vi "XNET Bus Monitor Example.vi"() -> ()   [LabVIEW 2025, in "XNET Bus Monitor Client.lvlib"]
uses:
  XNET Bus Monitor Client.lvlib
  Types/GUI.StateVariables.ctl
  Types/StreamEngine.CmdQueueData.ctl
  Types/StreamEngine.Parameters.ctl
  <vilib>/Utility/miscctls.llb/LVRowAndColumnUnsignedTypeDef.ctl
  Types/StreamEngine.CmdQueueData.Cmd.ctl
  Types/StreamEngine.QueueRefs.ctl
  Types/GUI.Controls.Refs.ctl
  bus_monitor_client/RPC Messages/ni_bus_monitor_api_Frame.ctl
  bus_monitor_client/bus_monitor_client.lvlib
  <vilib>/gRPC/LabVIEW gRPC Library/Shared/grpcId.ctl
  <vilib>/gRPC/LabVIEW gRPC Library/grpc-lvsupport-release.lvlib
  bus_monitor_client/RPC Messages/ni_bus_monitor_api_FrameFilter.ctl
  bus_monitor_client/RPC Messages/ni_bus_monitor_api_DirectionFilter.ctl
  bus_monitor_client/RPC Messages/ni_bus_monitor_api_FilterInfo.ctl
  bus_monitor_client/RPC Messages/ni_bus_monitor_api_SetStreamingFilterRequest.ctl
  bus_monitor_client/RPC Messages/ni_bus_monitor_api_PassThruRequest.ctl
  Types/gRPC.ConnectionInfo.ctl
  Types/StreamEngine.State.ctl
  Types/SubProcessEngine.CmdQueueData.ctl
  Types/SubProcessEngine.CmdQueueData.Cmd.ctl
  Types/SubProcessEngine.State.ctl
  bus_monitor_client/RPC Messages/ni_bus_monitor_api_ErrorInfo.ctl
  bus_monitor_client/RPC Messages/ni_bus_monitor_api_StreamBusReply.ctl
  Types/StreamEngine.CmdQueueData.InitialSettings.ctl
  Types/SubProcessEngine.CmdQueueData.Publish.ctl
  Types/SubProcessEngine.QueueRefs.ctl
  bus_monitor_client/RPC Messages/ni_bus_monitor_api_Session.ctl
  bus_monitor_client/RPC Messages/ni_bus_monitor_api_ResetStreamingFilterRequest.ctl
  bus_monitor_client/RPC Messages/ni_bus_monitor_api_GetStreamingFilterRequest.ctl
  bus_monitor_client/RPC Messages/ni_bus_monitor_api_StopProcessRequest.ctl
  bus_monitor_client/RPC Messages/ni_bus_monitor_api_LastCommError.ctl
  bus_monitor_client/RPC Messages/ni_bus_monitor_api_CommState.ctl
  bus_monitor_client/RPC Messages/ni_bus_monitor_api_CanCommState.ctl
panel:
  out "error out":errorcluster
  out "Device":string
  in  "Tab Control":enum32{"Bus Stream", "RAW"}(tab)
  out "Log Status":string
  in  "Direction Filter":T1
  in  "Type Filter":T2
  in  "Reset Filter":bool
  in  "Host Filter":bool
  in  "Filter IDs":string caption="Filter IDs (format = x<ID>, comma separated, ID x0 = Bus Error)"
  in  "Clear History":bool
  out "Table Control":string[][](table)
  in  "Sort By ID":bool
  out "Stream Connected":bool
  out "Bus Status":string
  in  "Log":bool
  in  "Pause":bool
  in  "Extended?":bool
  in  "Identifier":u32 format="%x"
  in  "Raw Bytes":u8[](array[numeric])
  in  "Type":T3(ring)
  out "Error":errorcluster
  in  "Clear Raw":bool
  in  "Send Raw":bool
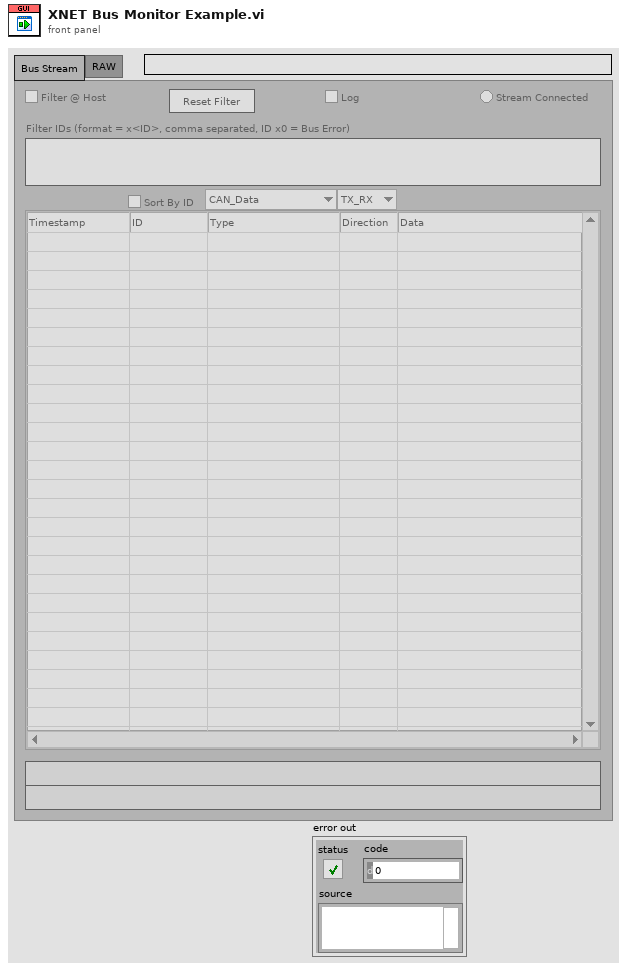
[diagram p1: front panel]
types:
  T1 = typedef "bus_monitor_client.lvlib/ni_bus_monitor_api_DirectionFilter.ctl" = enum32{"TX_RX", "RX", "TX"}
  T2 = typedef "bus_monitor_client.lvlib/ni_bus_monitor_api_FrameFilter.ctl" = enum32{"CAN_Data", "CAN_Remote", "CAN_Bus_Error", "CAN_2_Data", "CAN_FD_Data", "CAN_FD_BRS_Data", "J1939_Data", "Delay", "Log_Trigger", "Start_Trigger", "All"}
  T3 = enum16{"CAN Data", "CAN Remote", "CAN Bus Error", "CAN 2.0 Data", "CAN FD Data", "CAN FD+BRS Data", "J1939 Data", "Delay", "Log Trigger", "Start Trigger"}
  T4 = typedef "XNET Bus Monitor Client.lvlib/StreamEngine.CmdQueueData.InitialSettings.ctl" = cluster{"gRPC ID":T5, "Session":T6, "Project Folder":path}
  T5 = typedef "grpc-lvsupport-release.lvlib/grpcId.ctl" = u64
  T6 = typedef "bus_monitor_client.lvlib/ni_bus_monitor_api_Session.ctl" = cluster{"name":string, "session_uid":string}
  T7 = typedef "XNET Bus Monitor Client.lvlib/SubProcessEngine.State.ctl" = enum8{"Idle", "Arm", "Process", "Stop", "Exit"}
  T8 = typedef "XNET Bus Monitor Client.lvlib/StreamEngine.State.ctl" = enum8{"Wait", "Start Stream", "Read Stream", "Stop Stream", "Exit"}
  T9 = typedef "XNET Bus Monitor Client.lvlib/GUI.StateVariables.ctl" = cluster{"UI.Refs":T10, "Connected?":bool, "Stream.Qs":T11, "Log Path":path, "gRPC Info":T13}
  T10 = typedef "XNET Bus Monitor Client.lvlib/GUI.Controls.Refs.ctl" = cluster{"Device":refnum<vi>, "Pause":refnum<vi>, "Table Control":refnum<vi>, "Sort By ID":refnum<vi>, "Streaming Connected":refnum<vi>, "Bus Status":refnum<vi>, "Direction Filter":refnum<vi>, "Type Filter":refnum<vi>, "Clear History":refnum<vi>, "Filter IDs":refnum<vi>, "Filter Location":refnum<vi>, "Reset Filter":refnum<vi>, "Log":refnum<vi>, "Type":refnum<vi>, "Extended?":refnum<vi>, "Identifier":refnum<vi>, "Raw Bytes":refnum<vi>, "Send Raw":refnum<vi>, "Clear Raw":refnum<vi>, "Raw Error":refnum<vi>, "Log Status":refnum<vi>}
  T11 = typedef "XNET Bus Monitor Client.lvlib/StreamEngine.QueueRefs.ctl" = cluster{"Cmd":refnum<queue>, "SubProcesses":T12}
  T12 = typedef "XNET Bus Monitor Client.lvlib/SubProcessEngine.QueueRefs.ctl" = cluster{"Process":refnum<queue>, "Log":refnum<queue>}
  T13 = typedef "XNET Bus Monitor Client.lvlib/gRPC.ConnectionInfo.ctl" = cluster{"IP Address":string, "Service Name":string, "Found Port":u64, "ID":T5, "Session":T6}
  T14 = typedef "bus_monitor_client.lvlib/ni_bus_monitor_api_StopProcessRequest.ctl" = cluster{"session":T6}
  T15 = typedef "bus_monitor_client.lvlib/ni_bus_monitor_api_PassThruRequest.ctl" = cluster{"session":T6, "frame":T16}
  T16 = typedef "bus_monitor_client.lvlib/ni_bus_monitor_api_Frame.ctl" = cluster{"timestamp":dbl, "payload":u8[], "identifier":u32, "frame_type":u32, "extended":bool, "echo":bool}
  T17 = typedef "bus_monitor_client.lvlib/ni_bus_monitor_api_SetStreamingFilterRequest.ctl" = cluster{"session":T6, "filter_info":T18}
  T18 = typedef "bus_monitor_client.lvlib/ni_bus_monitor_api_FilterInfo.ctl" = cluster{"filter_ids":u32[], "direction_filter":T1, "frame_filter":T2}
  T19 = typedef "bus_monitor_client.lvlib/ni_bus_monitor_api_ResetStreamingFilterRequest.ctl" = cluster{"session":T6}
  T20 = typedef "bus_monitor_client.lvlib/ni_bus_monitor_api_GetStreamingFilterRequest.ctl" = cluster{"session":T6}
  T21 = typedef "LVRowAndColumnUnsignedTypeDef.ctl" = cluster{"Row":u32, "Column":u32}
  T22 = typedef "bus_monitor_client.lvlib/ni_bus_monitor_api_StopProcessReply.ctl" = cluster{"stopped":bool, "error":T23}
  T23 = typedef "bus_monitor_client.lvlib/ni_bus_monitor_api_ErrorInfo.ctl" = errorcluster
  T24 = enum8{"Enabled", "Disabled", "Disabled and Grayed Out"}
  T25 = typedef "bus_monitor_client.lvlib/ni_bus_monitor_api_PassThruReply.ctl" = cluster{"error":T23}
  T26 = typedef "bus_monitor_client.lvlib/ni_bus_monitor_api_SetStreamingFilterReply.ctl" = cluster{"error":T23}
  T27 = typedef "bus_monitor_client.lvlib/ni_bus_monitor_api_ResetStreamingFilterReply.ctl" = cluster{"filter_info":T18, "error":T23}
  T28 = typedef "bus_monitor_client.lvlib/ni_bus_monitor_api_GetStreamingFilterReply.ctl" = cluster{"filter_info":T18, "error":T23}
  T29 = typedef "XNET Bus Monitor Client.lvlib/SubProcessEngine.CmdQueueData.Publish.ctl" = cluster{"Response Data":T30, "Success":bool}
  T30 = typedef "bus_monitor_client.lvlib/ni_bus_monitor_api_StreamBusReply.ctl" = cluster{"can_comm_state":T31, "frame":T16[], "error":T23}
  T31 = typedef "bus_monitor_client.lvlib/ni_bus_monitor_api_CanCommState.ctl" = cluster{"fault_code":i32, "fault":bool, "comm_state":T32, "last_comm_error":T33, "receive_error_counter":u32, "transmit_error_counter":u32, "transceiver_error":bool, "sleep":bool}
  T32 = typedef "bus_monitor_client.lvlib/ni_bus_monitor_api_CommState.ctl" = enum32{"Error_Active", "Error_Passive", "Bus_Off", "Init"}
  T33 = typedef "bus_monitor_client.lvlib/ni_bus_monitor_api_LastCommError.ctl" = enum32{"None", "Stuff", "Form", "ACK", "Bit1", "Bit0", "CRC"}
  T34 = typedef "XNET Bus Monitor Client.lvlib/SubProcessEngine.CmdQueueData.ctl" = cluster{"Cmd":T35, "Parameters":variant}
  T35 = typedef "XNET Bus Monitor Client.lvlib/SubProcessEngine.CmdQueueData.Cmd.ctl" = enum16{"Arm", "Publish", "Stop", "Exit"}
  T36 = typedef "XNET Bus Monitor Client.lvlib/StreamEngine.Parameters.ctl" = cluster{"Host Filter":bool, "Filter Parameters":T18, "Sort By ID":bool, "Pause":bool, "Clear History":bool}
  T37 = typedef "XNET Bus Monitor Client.lvlib/StreamEngine.CmdQueueData.ctl" = cluster{"Cmd":T38, "Parameters":variant}
  T38 = typedef "XNET Bus Monitor Client.lvlib/StreamEngine.CmdQueueData.Cmd.ctl" = enum8{"Start Stream", "Stop Stream", "Exit"}
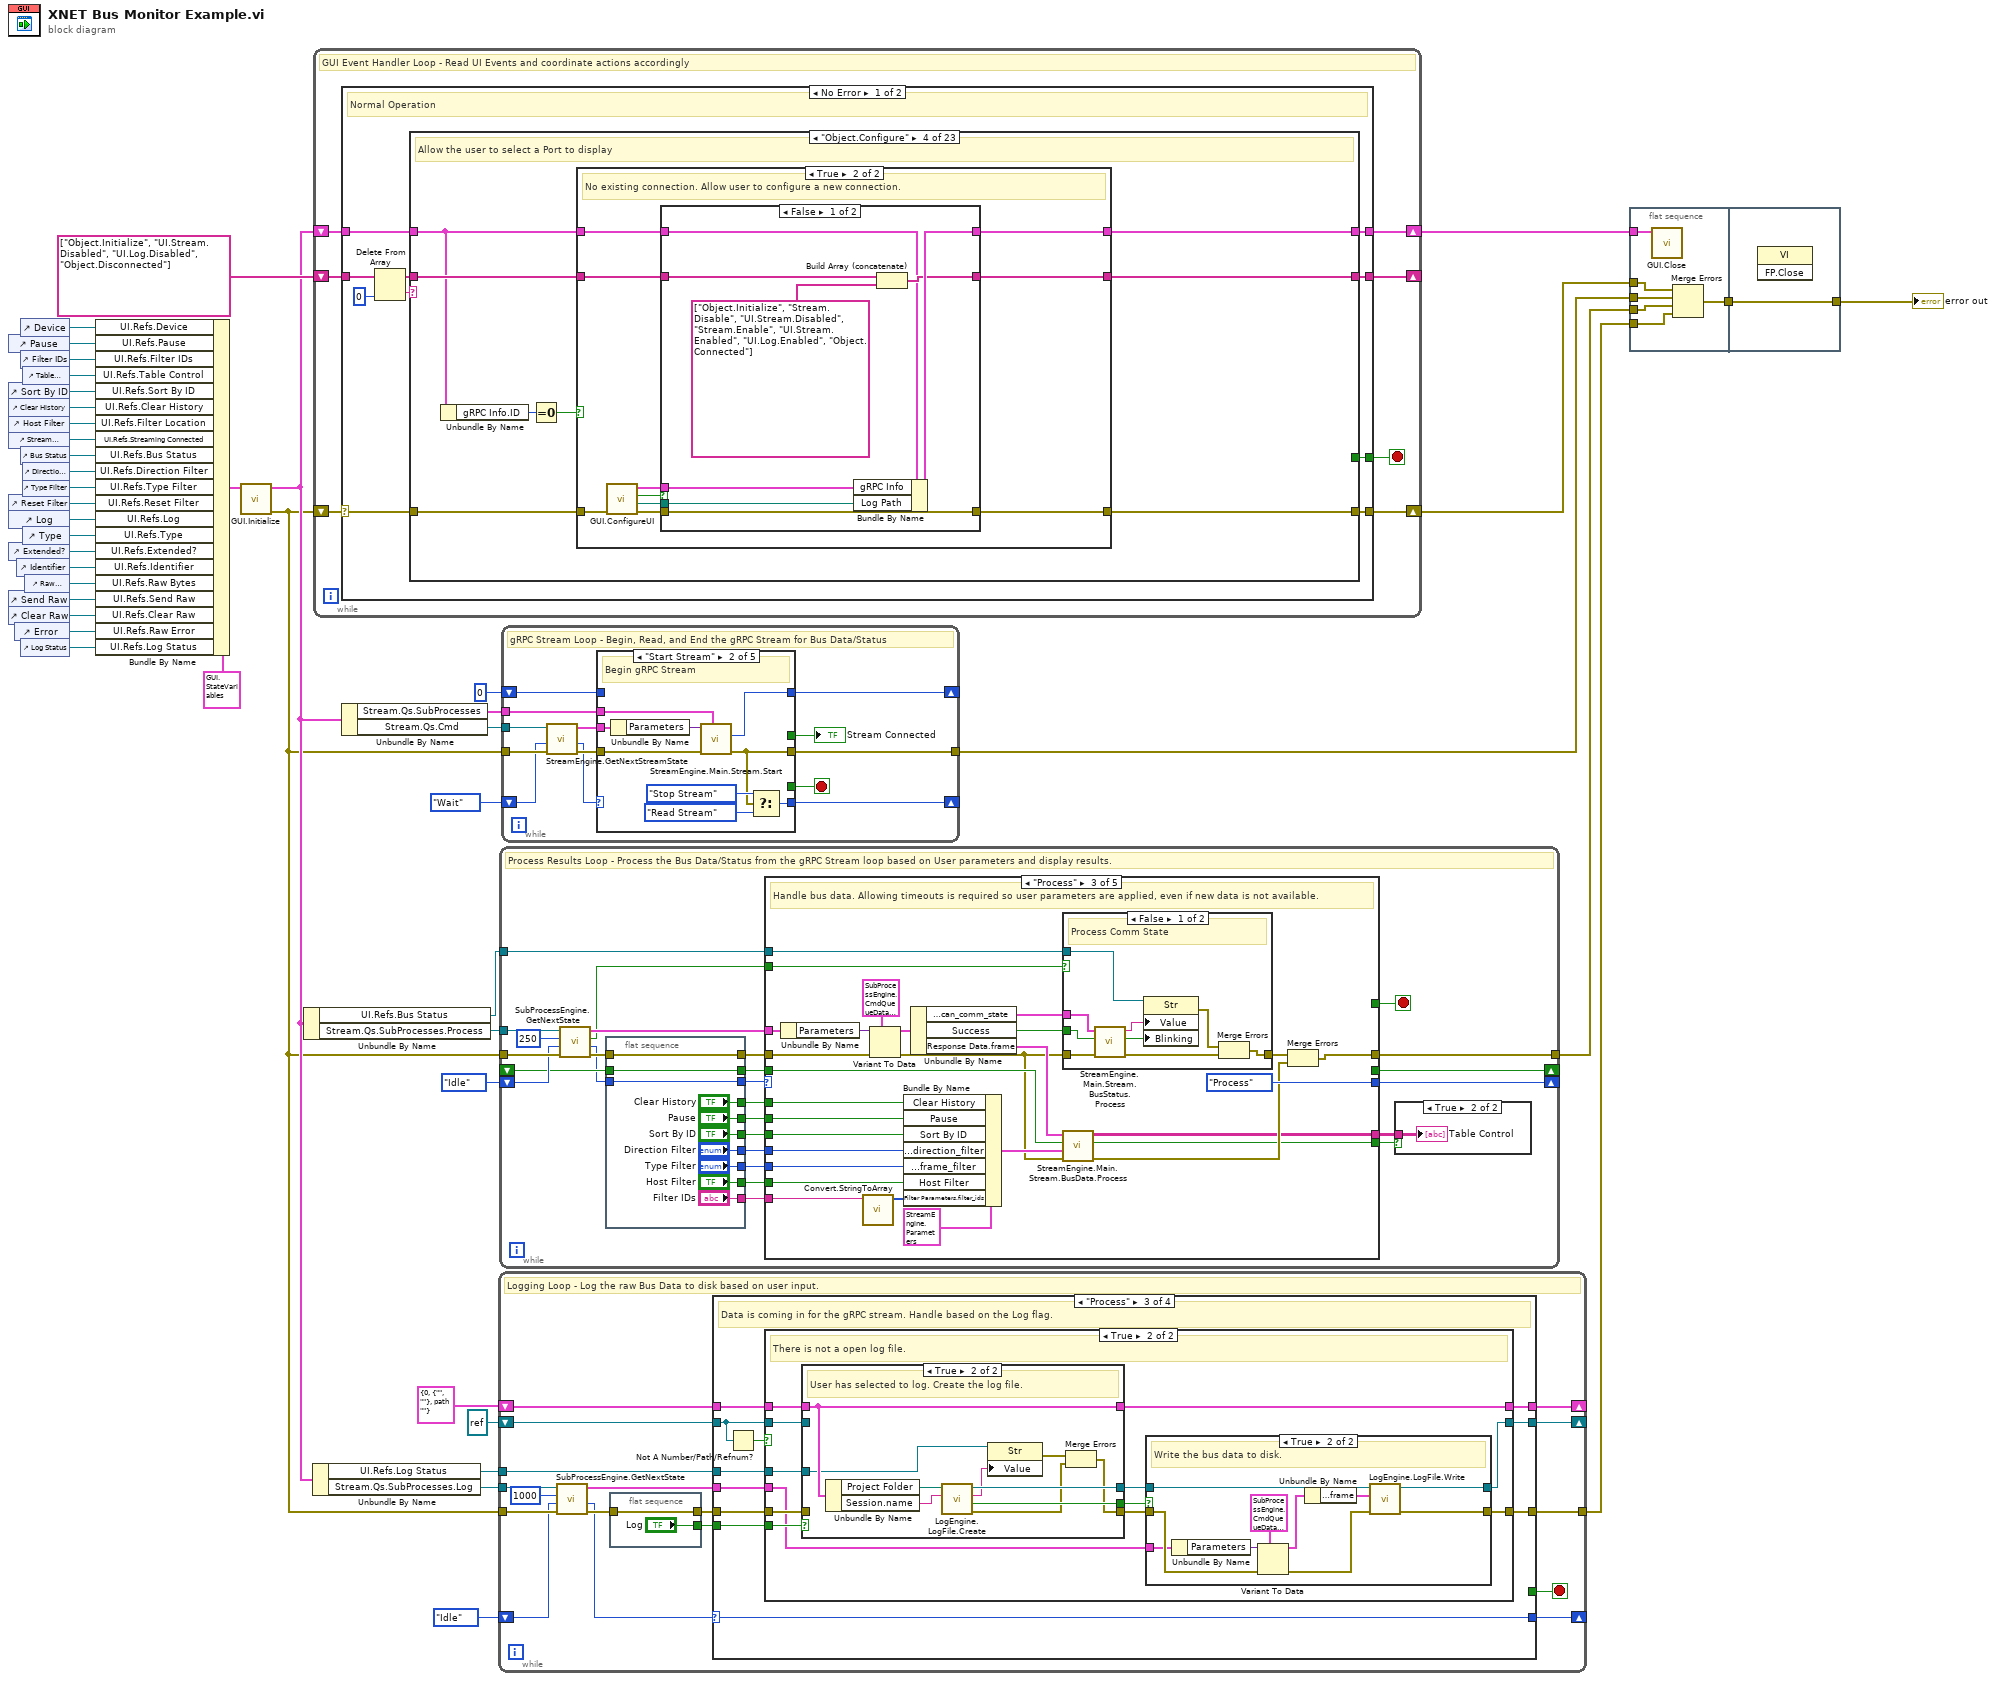
[diagram p0: block diagram]
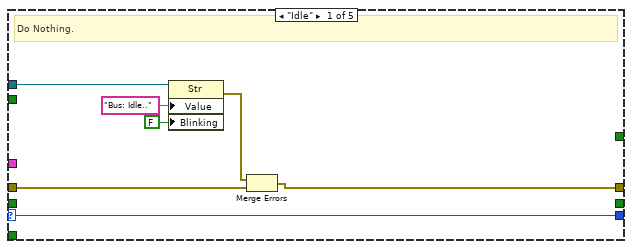
[diagram p3: hidden frame]
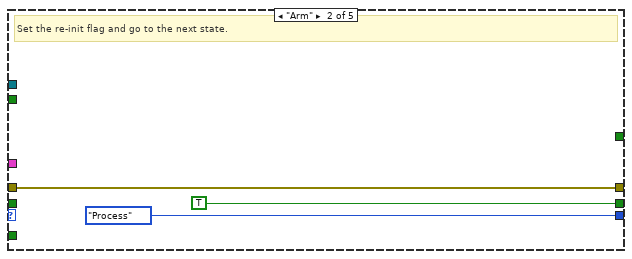
[diagram p4: hidden frame]
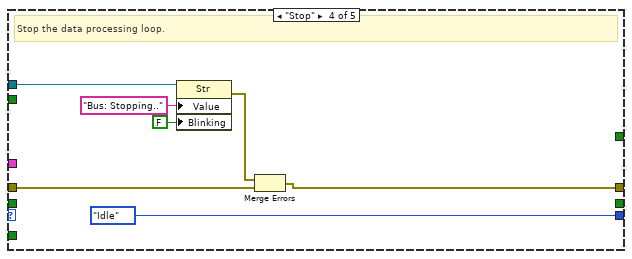
[diagram p6: hidden frame]
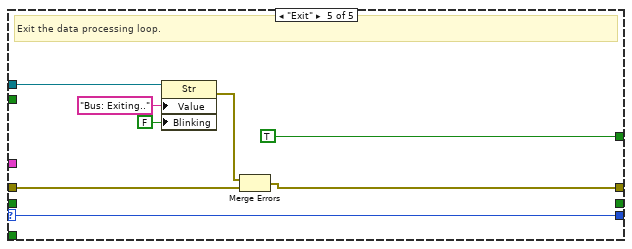
[diagram p7: hidden frame]
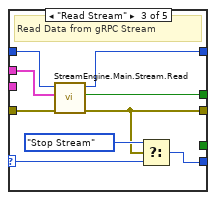
[diagram p9: hidden frame]
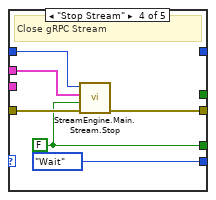
[diagram p10: hidden frame]
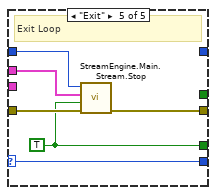
[diagram p11: hidden frame]
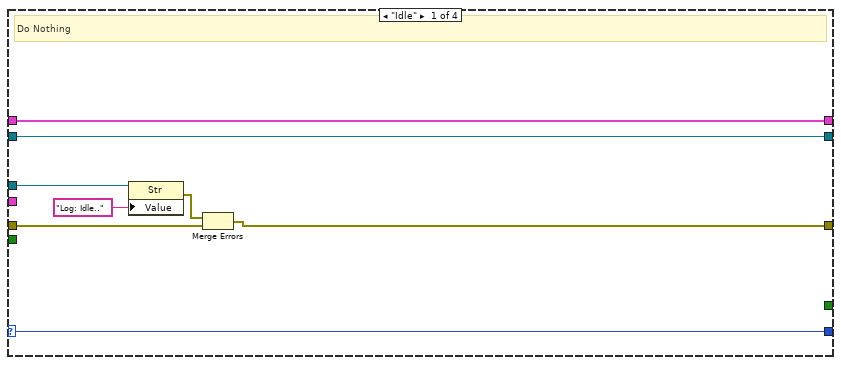
[diagram p12: hidden frame]
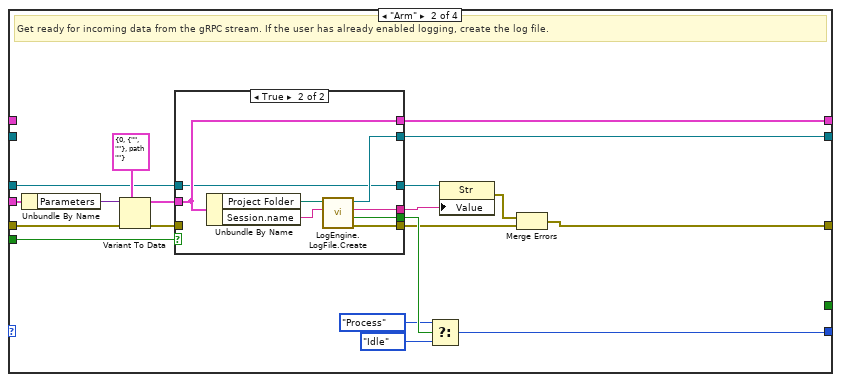
[diagram p13: hidden frame]
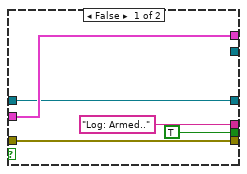
[diagram p14: hidden frame]
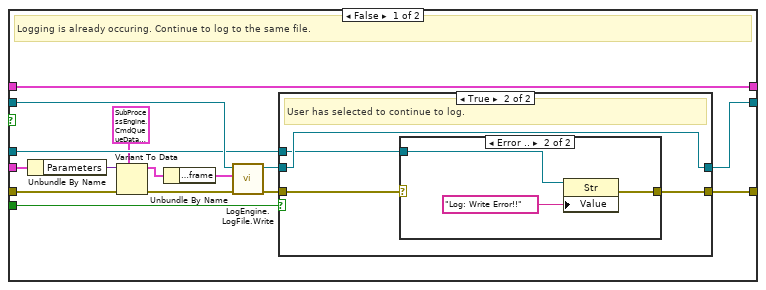
[diagram p15: hidden frame]
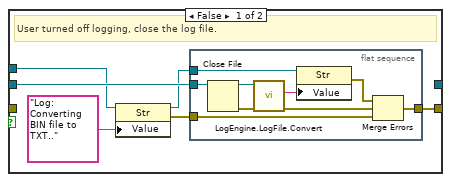
[diagram p16: hidden frame]
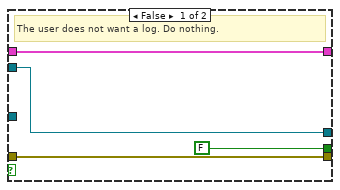
[diagram p19: hidden frame]
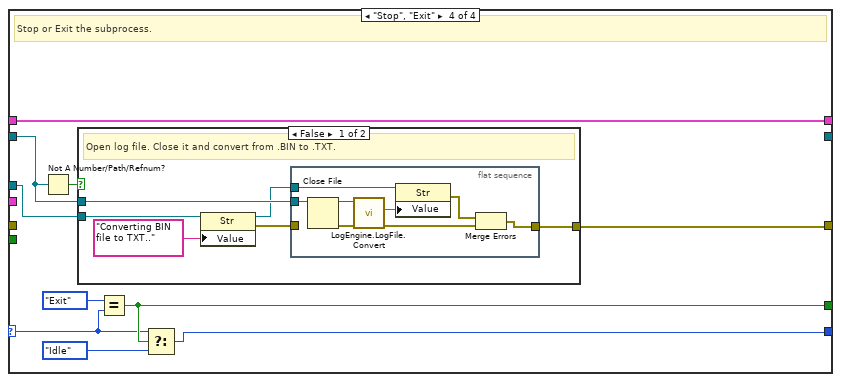
[diagram p20: hidden frame]
diagram:
  n1 = control-ref of="Pause"() -> (w22:refnum<vi>)
  n2 = control-ref of="Sort By ID"() -> (w41:refnum<vi>)
  n3 = control-ref of="Clear History"() -> (w37:refnum<vi>)
  n4 = control-ref of="Host Filter"() -> (w36:refnum<vi>)
  n5 = control-ref of="Stream Connected"() -> (w40:refnum<vi>)
  n6 = control-ref of="Reset Filter"() -> (w35:refnum<vi>)
  n7 = control-ref of="Log"() -> (w34:refnum<vi>)
  n8 = control-ref of="Extended?"() -> (w30:refnum<vi>)
  n9 = control-ref of="Send Raw"() -> (w27:refnum<vi>)
  n10 = control-ref of="Clear Raw"() -> (w28:refnum<vi>)
  n11 = control-ref of="Error"() -> (w29:refnum<vi>)
  n12 = control-ref of="Identifier"() -> (w31:refnum<vi>)
  n13 = control-ref of="Device"() -> (w24:refnum<vi>)
  n14 = control-ref of="Filter IDs"() -> (w38:refnum<vi>)
  n15 = control-ref of="Bus Status"() -> (w39:refnum<vi>)
  n16 = control-ref of="Log Status"() -> (w6:refnum<vi>)
  n17 = control-ref of="Table Control"() -> (w42:refnum<vi>)
  n18 = control-ref of="Direction Filter"() -> (w25:refnum<vi>)
  n19 = control-ref of="Type Filter"() -> (w26:refnum<vi>)
  n20 = control-ref of="Type"() -> (w33:refnum<vi>)
  n21 = control-ref of="Raw Bytes"() -> (w32:refnum<vi>)
  n22 = Bundle By Name(cluster=T9 {"UI.Refs"={"Device"=refnum, "Pause"=refnum, "Table Control"=refnum, "Sort By ID"=refnum, "Streaming Connected"=refnum, "Bus Status"=refnum, "Direction Filter"=refnum, "Type Filter"=refnum, "Clear History"=refnum, "Filter IDs"=refnum, "Filter Location"=refnum, "Reset Filter"=refnum, "Log"=refnum, "Type"=refnum, "Extended?"=refnum, "Identifier"=refnum, "Raw Bytes"=refnum, "Send Raw"=refnum, "Clear Raw"=refnum, "Raw Error"=refnum, "Log Status"=refnum}, "Connected?"=FALSE, "Stream.Qs"={"Cmd"=refnum, "SubProcesses"={"Process"=refnum, "Log"=refnum}}, "Log Path"=path "", "gRPC Info"={"IP Address"="", "Service Name"="", "Found Port"=0, "ID"=0, "Session"={"name"="", "session_uid"=""}}}, "UI.Refs.Device"=w24, "UI.Refs.Pause"=w22, "UI.Refs.Filter IDs"=w38, "UI.Refs.Table Control"=w42, "UI.Refs.Sort By ID"=w41, "UI.Refs.Clear History"=w37, "UI.Refs.Filter Location"=w36, "UI.Refs.Streaming Connected"=w40, "UI.Refs.Bus Status"=w39, "UI.Refs.Direction Filter"=w25, "UI.Refs.Type Filter"=w26, "UI.Refs.Reset Filter"=w35, "UI.Refs.Log"=w34, "UI.Refs.Type"=w33, "UI.Refs.Extended?"=w30, "UI.Refs.Identifier"=w31, "UI.Refs.Raw Bytes"=w32, "UI.Refs.Send Raw"=w27, "UI.Refs.Clear Raw"=w28, "UI.Refs.Raw Error"=w29, "UI.Refs.Log Status"=w6) -> (w23:T9)
  n23 = call "GUI.Initialize.vi"("State Variables in"=w23) -> ("error out"=w10:errorcluster, "State Variables out"=w13:T9)  [unwired: 9 in]
  n24 = Unbundle By Name(w13) -> ("UI.Refs.Bus Status"=w17:refnum<vi>, "Stream.Qs.SubProcesses.Process"=w18:refnum<queue>)
  n25 = Unbundle By Name(w13) -> ("UI.Refs.Log Status"=w5:refnum<vi>, "Stream.Qs.SubProcesses.Log"=w12:refnum<queue>)
  n26 = while {
    shift-right: [w50] -> _
    shift-left: string[] ["Object.Initialize", "UI.Stream.Disabled", "UI.Log.Disabled", "Object.Disconnected"] -> [w51]
    shift-right: [w48] -> w43
    shift-left: w13 -> [w47]
    shift-right: [w49] -> w8
    shift-left: w10 -> [w46]
    stop <- w52 stop-if-true
    # "GUI Event Handler Loop - Read UI Events and coordinate actions accordingly"
    n27 = case shown="No Error" w46 {
      selector: w46 -> [w53 w415]
      tunnel: [w62 _] -> w52
      tunnel: w51 -> [w60 w419]
      tunnel: [w57 w419] -> w50
      tunnel: [w56 w416] -> w49
      tunnel: [w55 w418] -> w48
      tunnel: w47 -> [w54 w418]
      frame No Error {
        # "Normal Operation"
        n28 = Delete From Array(array=w60, index=0) -> (deleted portion=w59:string, array with subset deleted=w58:string[])  [unwired: 1 in]
        n29 = case shown="\"Object.Configure\"" w59 {
          tunnel: [_ _ _ _ _ _ _ _ _ _ _ _ _ _ _ _ _ _ _ _ _ FALSE TRUE] -> w62
          tunnel: [w65 w71 w170 w178 w227 w236 w262 w264 w271 w285 w298 w311 w329 w333 w340 w354 w364 w379 w393 w399 w404 w410 w414] -> w57
          tunnel: w53 -> [w64 w69 w166 w176 w224 w233 w260 w266 w269 w282 w296 w308 w328 w332 w339 w352 w362 w377 w391 w394 w400 w407 w411]
          tunnel: w58 -> [w65 w70 w170 w177 w227 w236 w262 w263 w271 w285 w298 w311 w329 w333 w340 w354 w364 w379 w393 w399 w404 w410 w414]
          tunnel: w54 -> [w63 w66 w169 w174 w225 w230 w259 w267 w268 w284 w297 w310 w327 w331 w337 w353 w363 w378 w392 w398 w403 w406 w412]
          tunnel: [w64 w68 w162 w175 w214 w232 w250 w266 w270 w273 w295 w300 w328 w332 w338 w352 w362 w377 w391 w395 w401 w408 w411] -> w56
          tunnel: [w63 w67 w169 w179 w221 w231 w254 w267 w268 w284 w297 w310 w327 w331 w337 w353 w363 w378 w392 w398 w403 w406 w412] -> w55
          frame Default {
            # "Do nothing."
          }
          frame "" {
            # "Check for new events."
            n30 = event shown="[9] Panel Close?" {
              selector: _ -> [_ _ _ _ _ _ _ _ _ _]
              dyn-events: _ -> [_ _ _ _ _ _ _ _ _ _]
              timeout: 250 -> [_ _ _ _ _ _ _ _ _ _]
              tunnel: [w73 w78 w87 w99 w110 w119 w129 w142 w151 w158] -> w71
              tunnel: w70 -> [w73 w79 w88 w98 w109 w118 w128 w141 w152 w159]
              tunnel: w69 -> [w75 w80 w89 w100 w111 w120 w130 w143 w155 w161]
              tunnel: [w75 w80 w89 w100 w111 w120 w130 w143 w155 w161] -> w68
              tunnel: [w74 w77 w86 w97 w108 w117 w127 w140 w154 w160] -> w67
              tunnel: w66 -> [w74 w77 w86 w97 w108 w117 w127 w140 w154 w160]
              event Timeout {
                # "No new events to be handled. Do Nothing."
                n31 = event-data() -> ()  [unwired: 2 out]
              }
              event "Send Raw": Value Change {
                # "User entered a new raw message and is ready to Send."
                n32 = event-data() -> ()  [unwired: 2 out]
                n33 = Unbundle By Name(w77) -> ("Connected?"=w76:bool)
                n34 = case shown="True" w76 {
                  tunnel: w79 -> [w81 w83]
                  tunnel: [w81 w82] -> w78
                  frame False {
                  }
                  frame True {
                    n35 = Build Array (concatenate)(w83, string[] ["Raw.Send"]) -> (w82:string[])
                  }
                }
              }
              event "Clear Raw": Value Change {
                # "The user has selected to clear all the values in the Raw tab."
                n36 = event-data() -> ()  [unwired: 2 out]
                n37 = Unbundle By Name(w86) -> ("Connected?"=w85:bool)
                n38 = case shown="True" w85 {
                  tunnel: w88 -> [w90 w92]
                  tunnel: [w90 w91] -> w87
                  frame False {
                  }
                  frame True {
                    n39 = Build Array (concatenate)(w92, string[] ["Raw.Clear"]) -> (w91:string[])
                  }
                }
              }
              event "Filter IDs": Value Change {
                # "The user has changed which IDs to filter. Apply changes."
                n40 = event-data() -> ()  [unwired: 2 out]
                n41 = Unbundle By Name(w97) -> ("Connected?"=w95:bool)
                n42 = local read "Host Filter"() -> (w96:bool)
                n43 = Compound Arithmetic op=AND(invert w96, w95) -> (w94:bool)
                n44 = case shown="False" w94 {
                  tunnel: w98 -> [w101 w105]
                  tunnel: [w102 w104] -> w99
                  frame False {
                    # "Handle filtering on the client/host."
                    n45 = Build Array (concatenate)(w101, "Stream.Table.GoUp") -> (w102:string[])
                  }
                  frame True {
                    # "Send updated filter parameters to Server."
                    n46 = Build Array (concatenate)(w105, string[] ["Stream.Filter.Send", "Stream.Table.GoUp"]) -> (w104:string[])
                  }
                }
              }
              event "Clear History", "Sort By ID": Value Change {
                # "The user has selected to make table changes. The processing loop will handle this but make the table go to the top."
                n47 = event-data() -> ()  [unwired: 2 out]
                n48 = Unbundle By Name(w108) -> ("Connected?"=w107:bool)
                n49 = case shown="True" w107 {
                  tunnel: [w112 w115] -> w110
                  tunnel: w109 -> [w112 w114]
                  frame False {
                  }
                  frame True {
                    n50 = Build Array (concatenate)(w114, "Stream.Table.GoUp") -> (w115:string[])
                  }
                }
              }
              event "Reset Filter": Value Change {
                # "The user has reset which IDs to filter. Apply changes."
                n51 = event-data() -> ()  [unwired: 2 out]
                n52 = Unbundle By Name(w117) -> ("Connected?"=w116:bool)
                n53 = case shown="True" w116 {
                  tunnel: w118 -> [w121 w123]
                  tunnel: [w121 w122] -> w119
                  frame False {
                  }
                  frame True {
                    n54 = Build Array (concatenate)(w123, string[] ["Stream.Filter.Reset", "Stream.Table.GoUp"]) -> (w122:string[])
                  }
                }
              }
              event "Host Filter": Value Change {
                # "The user has changed where filtering happens. Apply changes."
                n55 = event-data() -> ("NewVal"=w125:bool)  [unwired: 1 out]
                n56 = Unbundle By Name(w127) -> ("Connected?"=w126:bool)
                n57 = case shown="True" w126 {
                  tunnel: w128 -> [w131 w134]
                  tunnel: [w131 w133] -> w129
                  tunnel: w125 -> [_ w132]
                  frame False {
                  }
                  frame True {
                    n58 = case shown="True" w132 {
                      tunnel: [string[] ["Stream.Filter.Send", "Stream.Table.GoUp"] string[] ["Stream.Filter.Clear", "Stream.Table.GoUp"]] -> w135
                      frame False {
                      }
                      frame True {
                      }
                    }
                    n59 = Build Array (concatenate)(w134, w135) -> (w133:string[])
                  }
                }
              }
              event "Log": Value Change {
                # "Log loop will handle the logging but force the GUI to latch the configuration while a log session is occuring."
                n60 = event-data() -> ("NewVal"=w138:bool)  [unwired: 1 out]
                n61 = Unbundle By Name(w140) -> ("Connected?"=w139:bool)
                n62 = case shown="True" w139 {
                  tunnel: w141 -> [w144 w147]
                  tunnel: [w144 w146] -> w142
                  tunnel: w138 -> [_ w145]
                  frame False {
                  }
                  frame True {
                    n63 = case shown="False" w145 {
                      tunnel: [string[] ["UI.Log.Disabled"] string[] ["UI.Log.Enabled"]] -> w148
                      frame False {
                      }
                      frame True {
                      }
                    }
                    n64 = Build Array (concatenate)(w147, w148) -> (w146:string[])
                  }
                }
              }
              event Menu Selection (User) {
                # "Queue up the Configure or Exit commands from the run time menu."
                n65 = event-data() -> ("ItemTag"=w153:string)  [unwired: 1 out]
                n66 = Build Array (concatenate)(w152, w153) -> (w151:string[])
              }
              event Panel Close? {
                # "Discard the user panel close and handle nicely."
                n67 = event-data() -> ()  [unwired: 5 out]
                n68 = Build Array (concatenate)(w159, "Object.Exit") -> (w158:string[])
                n69 = event-data("Discard?"=TRUE) -> ()  [unwired: 1 in, 1 out]
              }
            }
          }
          frame "Object.Initialize" {
            # "Initialize the GUI"
            n70 = Unbundle By Name(w169) -> ("UI.Refs.Device"=w164:refnum<vi>, "UI.Refs.Filter Location"=w167:refnum<vi>)
            n71 = property class="Bool (strict)"(reference=w167, error in=w166, "Value"=FALSE) -> (error out=w163:errorcluster)  [unwired: 1 out]
            n72 = local write "Tab Control"(0) -> ()
            n73 = property class="Str"(reference=w164, error in=w163, "Value"="Initializing!!") -> (error out=w162:errorcluster)  [unwired: 1 out]
          }
          frame "Object.Configure" {
            # "Allow the user to select a Port to display"
            n74 = Unbundle By Name(w174) -> ("gRPC Info.ID"=w173:T5)
            n75 = Equal To 0?(x=w173) -> (x = 0?=w172:bool)
            n76 = case shown="True" w172 {
              tunnel: [w181 w201] -> w179
              tunnel: [w180 w200] -> w178
              tunnel: w177 -> [w183 w199]
              tunnel: w176 -> [w187 w196]
              tunnel: [w187 w195] -> w175
              tunnel: w174 -> [w182 w192]
              frame False {
                # "A connection already exists. Ask the user if they want to close it."
                n77 = Two Button Dialog(message="Configuring will close the current session. Continue?", 2:"Yes" ("T button name (\"OK\")")) -> (T button?=w184:bool)  [unwired: 1 in]
                n78 = case shown="True" w184 {
                  tunnel: w183 -> [w188 _]
                  tunnel: w182 -> [w189 w191]
                  tunnel: [w189 w191] -> w181
                  tunnel: [w188 string[] ["Stream.Disable", "UI.Stream.Disabled", "UI.Log.Disabled", "Object.Disconnect", "Object.Disconnected", "Object.Initialize", "Object.Configure"]] -> w180
                  frame False {
                  }
                  frame True {
                  }
                }
              }
              frame True {
                # "No existing connection. Allow user to configure a new connection."
                n79 = call "GUI.ConfigureUI.vi"("error in (no error)"=w196) -> ("error out"=w194:errorcluster, "Log Path out"=w193:path, "Canceled?"=w198:bool, "gRPC Info"=w197:T13)  [unwired: 7 in]
                n80 = case shown="False" w198 {
                  tunnel: w192 -> [w204 w211]
                  tunnel: [w209 w211] -> w201
                  tunnel: [w207 w212] -> w200
                  tunnel: w199 -> [w208 w212]
                  tunnel: w197 -> [w205 _]
                  tunnel: [w203 w210] -> w195
                  tunnel: w194 -> [w203 w210]
                  tunnel: w193 -> [w202 _]
                  frame False {
                    n81 = Bundle By Name(cluster=w204, "gRPC Info"=w205, "Log Path"=w202) -> (w209:T9)
                    n82 = Build Array (concatenate)(w208, string[] ["Object.Initialize", "Stream.Disable", "UI.Stream.Disabled", "Stream.Enable", "UI.Stream.Enabled", "UI.Log.Enabled", "Object.Connected"]) -> (w207:string[])
                  }
                  frame True {
                    # "User canceled"
                  }
                }
              }
            }
          }
          frame "Object.Connected" {
            # "gRPC connected. Update the GUI accordingly."
            n83 = call "GUI.DisableState.Set.vi"("Enable?"=TRUE, "error in (no error)"=w224, "State Variables in"=w225) -> ("error out"=w220:errorcluster, "State Variables out"=w222:T9)  [unwired: 7 in]
            n84 = Unbundle By Name(w222) -> ("UI.Refs.Log"=w216:refnum<vi>, "Log Path"=w217:path, "UI.Refs.Device"=w219:refnum<vi>, "gRPC Info.Service Name"=w218:string)
            n85 = property class="Str"(reference=w219, error in=w220, "Value"=w218) -> (error out=w215:errorcluster)  [unwired: 1 out]
            n86 = call <vilib>:"Is Path and Not Empty.vi"("path"=w217) -> ("Is Path and Not Empty?"=w213:bool)  [unwired: 4 in]
            n87 = property class="Bool (strict)"(reference=w216, error in=w215, "Visible"=w213) -> (error out=w214:errorcluster)  [unwired: 1 out]
            n88 = Bundle By Name(cluster=w222, "Connected?"=TRUE) -> (w221:T9)
          }
          frame "Object.Disconnect" {
            # "Disconnect from the Server."
            n89 = Unbundle By Name(w230) -> ("gRPC Info.ID"=w234:T5, "gRPC Info.Session"=w228:T6)
            n90 = Bundle By Name(cluster=w230, "gRPC Info"=T13 {"IP Address"="", "Service Name"="", "Found Port"=0, "ID"=0, "Session"={"name"="", "session_uid"=""}}) -> (w231:T9)
            n91 = Equal To 0?(x=w234) -> (x = 0?=w235:bool)
            n92 = case shown="False" w235 {
              tunnel: w234 -> [w246 _]
              tunnel: w233 -> [w243 w248]
              tunnel: [w243 w248] -> w232
              tunnel: w228 -> [w237 _]
              frame False {
                n93 = Bundle By Name(cluster=T14 {"session"={"name"="", "session_uid"=""}} ("Request Data"), "session"=w237) -> (w238:T14)
                n94 = call "Bus_Monitor_API StopProcess.vi"("Request Data"=w238, "gRPC ID"=w246) -> ("error out"=w241:errorcluster, "Response Data"=w242:T22, "gRPC ID out"=w247:T5)  [unwired: 7 in]
                n95 = call "gRPC.Response.GetError.vi"("error in (no error)"=w241, "Response"=w242) -> ("error out"=w240:errorcluster)  [unwired: 9 in]
                n96 = call "Destroy Client.vi"("gRPC ID"=w247) -> ("error out"=w245:errorcluster)  [unwired: 10 in]
                n97 = Merge Errors(w240, w245) -> (w244:errorcluster)
                n98 = call <vilib>:"Simple Error Handler.vi"("error in (no error)"=w244) -> ()  [unwired: 4 in, 5 out]
              }
              frame True {
              }
            }
          }
          frame "Object.Disconnected" {
            # "Disconnected from the Server. Update the GUI accordingly."
            n99 = call "GUI.DisableState.Set.vi"("Enable?"=FALSE, "error in (no error)"=w260, "State Variables in"=w259) -> ("error out"=w256:errorcluster, "State Variables out"=w255:T9)  [unwired: 7 in]
            n100 = Unbundle By Name(w255) -> ("UI.Refs.Log"=w252:refnum<vi>, "UI.Refs.Device"=w257:refnum<vi>)
            n101 = property class="Str"(reference=w257, error in=w256, "Value"="Object Disconnected - Configure") -> (error out=w251:errorcluster)  [unwired: 1 out]
            n102 = property class="Bool (strict)"(reference=w252, error in=w251, "Visible"=TRUE ("Value")) -> (error out=w250:errorcluster)  [unwired: 1 out]
            n103 = Bundle By Name(cluster=w255, "Connected?"=FALSE) -> (w254:T9)
          }
          frame "Object.Exit" {
            # "Queue all the commands to cleanly exit."
            n104 = Build Array (concatenate)(w263, string[] ["Stream.Disable", "UI.Stream.Disabled", "UI.Log.Disabled", "Object.Disconnect", "Object.Disconnected", "Stream.Exit", "App.Exit"]) -> (w264:string[])
          }
          frame "UI.Stream.Enabled" {
            n105 = call "GUI.Stream.Enable.vi"("error in (no error)"=w269, "State Variables in"=w268) -> ("error out"=w270:errorcluster)  [unwired: 9 in]
          }
          frame "UI.Log.Enabled" {
            w272 = T24."Disabled and Grayed Out" ("Disabled")
            # "Logging has be enabled. Stop the user from changing filter settings so that the data coming from the Server is the same."
            n106 = Unbundle By Name(w284) -> ("UI.Refs.Type Filter"=w277:refnum<vi>, "UI.Refs.Filter IDs"=w276:refnum<vi>, "UI.Refs.Direction Filter"=w275:refnum<vi>, "UI.Refs.Reset Filter"=w280:refnum<vi>, "UI.Refs.Filter Location"=w283:refnum<vi>)
            n107 = property class="Bool (strict)"(reference=w283, error in=w282, "DisabledEnum"=w272) -> (error out=w281:errorcluster, "Value"=w279:bool)  [unwired: 1 out]
            n108 = Build Array(w277, w276, w275) -> (w274:refnum<vi>[])
            n109 = property class="Bool"(reference=w280, error in=w281, "DisabledEnum"=w272) -> (error out=w278:errorcluster)  [unwired: 1 out]
            n110 = case shown="False" w279 {
              tunnel: w278 -> [w288 w294]
              tunnel: w274 -> [w289 _]
              tunnel: [w287 w294] -> w273
              tunnel: w272 -> [w286 _]
              frame False {
                n111 = for {
                  tunnel: w289 -> [w293] mode=indexing
                  shift-right: [w291] -> w287
                  shift-left: w288 -> [w292]
                  tunnel: w286 -> [w290]
                  n112 = property class="Ctl"(reference=w293, error in=w292, "DisabledEnum"=w290) -> (error out=w291:errorcluster)  [unwired: 1 out]
                }
              }
              frame True {
              }
            }
          }
          frame "UI.Stream.Disabled" {
            n113 = call "GUI.Stream.Disable.vi"("error in (no error)"=w296, "State Variables in"=w297) -> ("error out"=w295:errorcluster)  [unwired: 9 in]
          }
          frame "UI.Log.Disabled" {
            w299 = T24."Enabled" ("Disabled")
            # "Logging has been turned off so re-enable the filter options."
            n114 = Unbundle By Name(w310) -> ("UI.Refs.Type Filter"=w304:refnum<vi>, "UI.Refs.Filter IDs"=w303:refnum<vi>, "UI.Refs.Direction Filter"=w302:refnum<vi>, "UI.Refs.Reset Filter"=w306:refnum<vi>, "UI.Refs.Filter Location"=w309:refnum<vi>)
            n115 = property class="Bool (strict)"(reference=w309, error in=w308, "DisabledEnum"=w299) -> (error out=w307:errorcluster)  [unwired: 1 out]
            n116 = Build Array(w304, w303, w302) -> (w301:refnum<vi>[])
            n117 = property class="Bool"(reference=w306, error in=w307, "DisabledEnum"=w299) -> (error out=w305:errorcluster)  [unwired: 1 out]
            n118 = for {
              tunnel: w301 -> [w315] mode=indexing
              shift-right: [w313] -> w300
              shift-left: w305 -> [w314]
              tunnel: w299 -> [w312]
              n119 = property class="Ctl"(reference=w315, error in=w314, "DisabledEnum"=w312) -> (error out=w313:errorcluster)  [unwired: 1 out]
            }
          }
          frame "Raw.Send" {
            # "Send a raw frame to be put directly on the bus."
            n120 = Unbundle By Name(w327) -> ("gRPC Info.ID"=w320:T5, "gRPC Info.Session"=w316:T6)
            n121 = Bundle By Name(cluster=T15 {"session"={"name"="", "session_uid"=""}, "frame"={"timestamp"=0.0, "payload"=[], "identifier"=0, "frame_type"=0, "extended"=FALSE, "echo"=FALSE}} ("Request Data"), "session"=w316, "frame.extended"="Extended?", "frame.frame_type"="Type", "frame.identifier"="Identifier", "frame.payload"="Raw Bytes") -> (w321:T15)
            n122 = call "Bus_Monitor_API PassThru.vi"("Request Data"=w321, "gRPC ID"=w320) -> ("error out"=w318:errorcluster, "Response Data"=w319:T25)  [unwired: 7 in, 1 out]
            n123 = call "gRPC.Response.GetError.vi"("error in (no error)"=w318, "Response"=w319) -> ("error out"=→"Error":errorcluster)  [unwired: 9 in]
          }
          frame "Raw.Clear" {
            # "Clear the raw bytes GUI."
            n124 = local write "Raw Bytes"(u8[] [] ("Cmd")) -> ()
          }
          frame "Stream.Enable" {
            # "Start the gRPC stream loop."
            n125 = Unbundle By Name(w337) -> ("Stream.Qs"=w336:T11, "gRPC Info"=w335:T13, "Log Path"=w334:path)  [unwired: 1 out]
            n126 = call "StreamEngine.StartCmd.Send.vi"("error in (no error)"=w339, "Project Folder"=w334, "gRPC Info"=w335, "Q Refs"=w336) -> ("error out"=w338:errorcluster)  [unwired: 7 in]
          }
          frame "Stream.Filter.Send" {
            # "Send a filter update to the server."
            n127 = Unbundle By Name(w353) -> ("gRPC Info.ID"=w345:T5, "gRPC Info.Session"=w341:T6)
            n128 = local read "Direction Filter"() -> (w350:T1)
            n129 = local read "Type Filter"() -> (w349:T2)
            n130 = local read "Filter IDs"() -> (w351:string)
            n131 = call "Convert.StringToArray.vi"("Filter IDs"=w351) -> ("Filter IDs"=w348:u32[])  [unwired: 10 in]
            n132 = Bundle By Name(cluster=T17 {"session"={"name"="", "session_uid"=""}, "filter_info"={"filter_ids"=[], "direction_filter"=enum."TX_RX", "frame_filter"=enum."CAN_Data"}} ("Request Data"), "session"=w341, "filter_info.frame_filter"=w349, "filter_info.direction_filter"=w350, "filter_info.filter_ids"=w348) -> (w346:T17)
            n133 = call "Bus_Monitor_API SetStreamingFilter.vi"("Request Data"=w346, "gRPC ID"=w345) -> ("error out"=w344:errorcluster, "Response Data"=w342:T26)  [unwired: 7 in, 1 out]
            n134 = call "gRPC.Response.GetError.vi"("error in (no error)"=w344, "Response"=w342) -> ("error out"=w343:errorcluster)  [unwired: 9 in]
            n135 = call <vilib>:"Simple Error Handler.vi"("error in (no error)"=w343) -> ()  [unwired: 4 in, 5 out]
          }
          frame "Stream.Filter.Clear" {
            # "Command the server to clear out the filters."
            n136 = Unbundle By Name(w363) -> ("gRPC Info.ID"=w360:T5, "gRPC Info.Session"=w355:T6)
            n137 = Bundle By Name(cluster=T17 {"session"={"name"="", "session_uid"=""}, "filter_info"={"filter_ids"=[], "direction_filter"=enum."TX_RX", "frame_filter"=enum."CAN_Data"}} ("Request Data"), "session"=w355) -> (w356:T17)
            n138 = call "Bus_Monitor_API SetStreamingFilter.vi"("Request Data"=w356, "gRPC ID"=w360) -> ("error out"=w358:errorcluster, "Response Data"=w359:T26)  [unwired: 7 in, 1 out]
            n139 = call "gRPC.Response.GetError.vi"("error in (no error)"=w358, "Response"=w359) -> ("error out"=w357:errorcluster)  [unwired: 9 in]
            n140 = call <vilib>:"Simple Error Handler.vi"("error in (no error)"=w357) -> ()  [unwired: 4 in, 5 out]
          }
          frame "Stream.Filter.Reset" {
            # "Send a command to the server to reset the filter back to the default configuration."
            n141 = Unbundle By Name(w378) -> ("gRPC Info.ID"=w371:T5, "gRPC Info.Session"=w365:T6)
            n142 = Bundle By Name(cluster=T19 {"session"={"name"="", "session_uid"=""}} ("Request Data"), "session"=w365) -> (w366:T19)
            n143 = call "Bus_Monitor_API ResetStreamingFilter.vi"("Request Data"=w366, "gRPC ID"=w371) -> ("error out"=w369:errorcluster, "Response Data"=w370:T27)  [unwired: 7 in, 1 out]
            n144 = Unbundle By Name(w370) -> ("filter_info.filter_ids"=w373:u32[], "filter_info.direction_filter"=w375:T1, "filter_info.frame_filter"=w374:T2)
            n145 = call "gRPC.Response.GetError.vi"("error in (no error)"=w369, "Response"=w370) -> ("error out"=w368:errorcluster)  [unwired: 9 in]
            n146 = call <vilib>:"Simple Error Handler.vi"("error in (no error)"=w368) -> ()  [unwired: 4 in, 5 out]
            n147 = local write "Host Filter"(FALSE ("Host Filter")) -> ()
            n148 = call "Convert.ArrayToString.vi"("Filter IDs"=w373) -> ("Filter IDs"=w372:string)  [unwired: 10 in]
            n149 = local write "Filter IDs"(w372) -> ()
            n150 = local write "Direction Filter"(w375) -> ()
            n151 = local write "Type Filter"(w374) -> ()
          }
          frame "Stream.Filter.Read" {
            # "Get the current filter settings from the Server."
            n152 = Unbundle By Name(w392) -> ("gRPC Info.ID"=w386:T5, "gRPC Info.Session"=w380:T6)
            n153 = Bundle By Name(cluster=T20 {"session"={"name"="", "session_uid"=""}} ("Request Data"), "session"=w380) -> (w381:T20)
            n154 = call "Bus_Monitor_API GetStreamingFilter.vi"("Request Data"=w381, "gRPC ID"=w386) -> ("error out"=w385:errorcluster, "Response Data"=w384:T28)  [unwired: 7 in, 1 out]
            n155 = Unbundle By Name(w384) -> ("filter_info.filter_ids"=w388:u32[], "filter_info.direction_filter"=w390:T1, "filter_info.frame_filter"=w389:T2)
            n156 = call "gRPC.Response.GetError.vi"("error in (no error)"=w385, "Response"=w384) -> ("error out"=w383:errorcluster)  [unwired: 9 in]
            n157 = call <vilib>:"Simple Error Handler.vi"("error in (no error)"=w383) -> ()  [unwired: 4 in, 5 out]
            n158 = call "Convert.ArrayToString.vi"("Filter IDs"=w388) -> ("Filter IDs"=w387:string)  [unwired: 10 in]
            n159 = local write "Filter IDs"(w387) -> ()
            n160 = local write "Direction Filter"(w390) -> ()
            n161 = local write "Type Filter"(w389) -> ()
          }
          frame "Stream.Table.GoUp" {
            # "Go to the top of the bus table. This is needed for when filters are applied and the user has scrolled down in the list."
            n162 = Unbundle By Name(w398) -> ("UI.Refs.Table Control"=w396:refnum<vi>)
            n163 = property class="Tbl (strict)"(reference=w396, error in=w394, "Index Values"=T21 {"Row"=0, "Column"=0}) -> (error out=w395:errorcluster)  [unwired: 1 out]
          }
          frame "Stream.Disable" {
            # "Stop the gRPC stream to the Server."
            n164 = Unbundle By Name(w403) -> ("Stream.Qs"=w402:T11)
            n165 = call "StreamEngine.StopCmd.Send.vi"("error in (no error)"=w400, "Q Refs"=w402) -> ("error out"=w401:errorcluster)  [unwired: 9 in]
          }
          frame "Stream.Exit" {
            # "Tell the gRPC stream loop to exit."
            n166 = Unbundle By Name(w406) -> ("Stream.Qs"=w405:T11)
            n167 = call "StreamEngine.ExitCmd.Send.vi"("error in (no error)"=w407, "Q Refs"=w405) -> ("error out"=w408:errorcluster)  [unwired: 9 in]
          }
          frame "App.Exit" {
            # "Stop the GUI Event Handler (this) Loop."
          }
        }
      }
      frame Error {
        # "Handle Errors."
        n168 = call <vilib>:"Simple Error Handler.vi"("error in (no error)"=w415) -> ("error out"=w417:errorcluster)  [unwired: 4 in, 4 out]
        n169 = call <vilib>:"Clear Errors.vi"("error in (no error)"=w417) -> ("error out"=w416:errorcluster)  [unwired: 5 in, 1 out]
      }
    }
  }
  n170 = Unbundle By Name(w13) -> ("Stream.Qs.SubProcesses"=w15:T12, "Stream.Qs.Cmd"=w20:refnum<queue>)
  n171 = while {
    tunnel: w12 -> [w436]
    shift-right: [w431] -> _
    shift-left: SubProcessEngine.State."Idle" ("State") -> [w422]
    tunnel: w10 -> [w435]
    shift-right: [w434] -> _
    shift-left: refnum<file> refnum ("Byte Stream File out") -> [w433]
    shift-right: [w429] -> _
    shift-left: T4 {"gRPC ID"=0, "Session"={"name"="", "session_uid"=""}, "Project Folder"=path ""} ("cluster") -> [w428]
    tunnel: [w424] -> w7
    tunnel: w5 -> [w423]
    stop <- w430 stop-if-true
    # "Logging Loop - Log the raw Bus Data to disk based on user input."
    n172 = call "SubProcessEngine.GetNextState.vi"("error in (no error)"=w435, "State"=w422, "timeout in ms (5)"=1000, "Q"=w436) -> ("error out"=w426:errorcluster, "State"=w420:T7, "Data"=w432:T34)  [unwired: 4 in, 1 out]
    n173 = flat-sequence {
      tunnel: ["Log"] -> w427
      tunnel: w426 -> [w437]
      tunnel: [w437] -> w425
      frame #0 {
      }
    }
    n174 = case shown="\"Process\"" w420 {
      selector: w420 -> [w445 _ w480 w567]
      tunnel: [w446 w458 w488 _] -> w434
      tunnel: w433 -> [w446 _ w487 w574]
      tunnel: [w440 w450 w489 w566] -> w424
      tunnel: w425 -> [w441 w462 w482 _]
      tunnel: w432 -> [_ w465 w481 _]
      tunnel: [w445 w454 w480 w568] -> w431
      tunnel: [_ _ _ w571] -> w430
      tunnel: [w444 w460 w485 w573] -> w429
      tunnel: w428 -> [w444 _ w486 w573]
      tunnel: w427 -> [_ w453 w484 _]
      tunnel: w423 -> [w443 w448 w479 w572]
      frame "Idle" {
        # "Do Nothing"
        n175 = property class="Str"(reference=w443, "Value"="Log: Idle..") -> (error out=w442:errorcluster)  [unwired: 1 in, 1 out]
        n176 = Merge Errors(w442, w441) -> (w440:errorcluster)
      }
      frame "Arm" {
        # "Get ready for incoming data from the gRPC stream. If the user has already enabled logging, create the log file."
        n177 = Unbundle By Name(w465) -> ("Parameters"=w464:variant)
        n178 = Variant To Data(error in=w462, type=T4 {"gRPC ID"=0, "Session"={"name"="", "session_uid"=""}, "Project Folder"=path ""} ("cluster"), Variant=w464) -> (data=w461:T4, error out=w459:errorcluster)
        n179 = case shown="True" w453 {
          tunnel: ["Log: Armed.." ("Status") w476] -> w451
          tunnel: [w470 w475] -> w449
          tunnel: w459 -> [w470 _]
          tunnel: [TRUE ("Continue") w474] -> w457
          tunnel: w461 -> [w468 w473]
          tunnel: [w468 w473] -> w460
          tunnel: [_ w472] -> w458
          tunnel: w448 -> [w466 w471]
          tunnel: [w466 w471] -> w447
          frame False {
          }
          frame True {
            n180 = Unbundle By Name(w473) -> ("Project Folder"=w478:path, "Session.name"=w477:string)
            n181 = call "LogEngine.LogFile.Create.vi"("Port"=w477, "Project Folder"=w478) -> ("error out"=w475:errorcluster, "Continue"=w474:bool, "Status"=w476:string, "Byte Stream File out"=w472:refnum<file>)  [unwired: 6 in]
          }
        }
        n182 = Select(t=SubProcessEngine.State."Process" ("State"), s=w457, f=SubProcessEngine.State."Idle") -> (s? t:f=w454:T7)
        n183 = property class="Str"(reference=w447, "Value"=w451) -> (error out=w452:errorcluster)  [unwired: 1 in, 1 out]
        n184 = Merge Errors(w452, w449) -> (w450:errorcluster)
      }
      frame "Process" {
        # "Data is coming in for the gRPC stream. Handle based on the Log flag."
        n185 = Not A Number/Path/Refnum?(number/path/refnum=w487) -> (NaN/Path/Refnum?=w483:bool)
        n186 = case shown="True" w483 {
          tunnel: [w491 w528] -> w489
          tunnel: [w492 w537] -> w488
          tunnel: w487 -> [w502 w536]
          tunnel: w486 -> [w504 w534]
          tunnel: [w504 w533] -> w485
          tunnel: w484 -> [w495 w532]
          tunnel: w482 -> [w503 w531]
          tunnel: w481 -> [w497 w530]
          tunnel: w479 -> [w493 w529]
          frame False {
            # "Logging is already occuring. Continue to log to the same file."
            n187 = Unbundle By Name(w497) -> ("Parameters"=w500:variant)
            n188 = Variant To Data(error in=w503, type=T29 {"Response Data"={"can_comm_state"={"fault_code"=0, "fault"=FALSE, "comm_state"=enum."Error_Active", "last_comm_error"=enum."None", "receive_error_counter"=0, "transmit_error_counter"=0, "transceiver_error"=FALSE, "sleep"=FALSE}, "frame"=[], "error"={"status"=FALSE, "code"=0, "source"=""}}, "Success"=FALSE} ("cluster"), Variant=w500) -> (data=w499:T29, error out=w501:errorcluster)
            n189 = Unbundle By Name(w499) -> ("Response Data.frame"=w498:T16[])
            n190 = call "LogEngine.LogFile.Write.vi"("error in (no error)"=w501, "Data"=w498, "Byte Stream File in"=w502) -> ("error out"=w494:errorcluster, "Byte Stream File out"=w496:refnum<file>)  [unwired: 7 in]
            n191 = case shown="True" w495 {
              tunnel: w496 -> [w510 w523]
              tunnel: [w506 w520] -> w491
              tunnel: w493 -> [w509 w522]
              tunnel: w494 -> [_ w521]
              tunnel: [_ w523] -> w492
              frame False {
                # "User turned off logging, close the log file."
                n192 = property class="Str"(reference=w509, "Value"="Log: Converting BIN file to TXT..") -> (reference out=w507:refnum<vi>, error out=w505:errorcluster)  [unwired: 1 in]
                n193 = flat-sequence {
                  tunnel: w510 -> [w519]
                  tunnel: w507 -> [w515]
                  tunnel: [w513] -> w506
                  tunnel: w505 -> [w511]
                  frame #0 {
                    n194 = Close File(refnum=w519) -> (path=w518:path, error out=w517:errorcluster)  [unwired: 1 in]
                    n195 = call "LogEngine.LogFile.Convert.vi"("error in (no error)"=w517, "path"=w518) -> ("error out"=w512:errorcluster, "Status"=w514:string)  [unwired: 8 in]
                    n196 = property class="Str"(reference=w515, "Value"=w514) -> (error out=w516:errorcluster)  [unwired: 1 in, 1 out]
                    n197 = Merge Errors(w516, w512, w511) -> (w513:errorcluster)
                  }
                }
              }
              frame True {
                # "User has selected to continue to log."
                n198 = case shown="Error .." w521 {
                  selector: w521 -> [w524 _]
                  tunnel: w522 -> [_ w527]
                  tunnel: [w524 w525] -> w520
                  frame No Error {
                  }
                  frame Error {
                    n199 = property class="Str"(reference=w527, "Value"="Log: Write Error!!") -> (error out=w525:errorcluster)  [unwired: 1 in, 1 out]
                  }
                }
              }
            }
          }
          frame True {
            # "There is not a open log file."
            n200 = case shown="True" w532 {
              tunnel: [w554 w556] -> w539
              tunnel: [w555 w563] -> w538
              tunnel: w536 -> [w555 _]
              tunnel: [FALSE ("Continue") w562] -> w535
              tunnel: w531 -> [w554 _]
              tunnel: w534 -> [w553 w561]
              tunnel: [w553 w561] -> w533
              tunnel: w529 -> [_ w559]
              frame False {
                # "The user does not want a log. Do nothing."
              }
              frame True {
                # "User has selected to log. Create the log file."
                n201 = Unbundle By Name(w561) -> ("Project Folder"=w565:path, "Session.name"=w564:string)
                n202 = call "LogEngine.LogFile.Create.vi"("Port"=w564, "Project Folder"=w565) -> ("error out"=w557:errorcluster, "Continue"=w562:bool, "Status"=w558:string, "Byte Stream File out"=w563:refnum<file>)  [unwired: 6 in]
                n203 = property class="Str"(reference=w559, "Value"=w558) -> (error out=w560:errorcluster)  [unwired: 1 in, 1 out]
                n204 = Merge Errors(w560, w557) -> (w556:errorcluster)
              }
            }
            n205 = case shown="True" w535 {
              tunnel: w539 -> [w540 w547]
              tunnel: w538 -> [w541 w551]
              tunnel: [w540 w550] -> w528
              tunnel: [w541 w549] -> w537
              tunnel: w530 -> [_ w546]
              frame False {
                # "Do nothing."
              }
              frame True {
                # "Write the bus data to disk."
                n206 = Unbundle By Name(w546) -> ("Parameters"=w545:variant)
                n207 = Variant To Data(error in=w547, type=T29 {"Response Data"={"can_comm_state"={"fault_code"=0, "fault"=FALSE, "comm_state"=enum."Error_Active", "last_comm_error"=enum."None", "receive_error_counter"=0, "transmit_error_counter"=0, "transceiver_error"=FALSE, "sleep"=FALSE}, "frame"=[], "error"={"status"=FALSE, "code"=0, "source"=""}}, "Success"=FALSE} ("cluster"), Variant=w545) -> (data=w544:T29, error out=w548:errorcluster)
                n208 = Unbundle By Name(w544) -> ("Response Data.frame"=w543:T16[])
                n209 = call "LogEngine.LogFile.Write.vi"("error in (no error)"=w548, "Data"=w543, "Byte Stream File in"=w551) -> ("error out"=w550:errorcluster, "Byte Stream File out"=w549:refnum<file>)  [unwired: 7 in]
              }
            }
          }
        }
      }
      frame "Stop", "Exit" {
        # "Stop or Exit the subprocess."
        n210 = Not A Number/Path/Refnum?(number/path/refnum=w574) -> (NaN/Path/Refnum?=w575:bool)
        n211 = case shown="False" w575 {
          tunnel: w574 -> [w581 _]
          tunnel: w572 -> [w580 _]
          tunnel: [w577 _] -> w566
          frame False {
            # "Open log file. Close it and convert from .BIN to .TXT."
            n212 = property class="Str"(reference=w580, "Value"="Converting BIN file to TXT..") -> (reference out=w578:refnum<vi>, error out=w576:errorcluster)  [unwired: 1 in]
            n213 = flat-sequence {
              tunnel: w581 -> [w588]
              tunnel: w578 -> [w585]
              tunnel: [w584] -> w577
              tunnel: w576 -> [_]
              frame #0 {
                n214 = Close File(refnum=w588) -> (path=w583:path, error out=w582:errorcluster)  [unwired: 1 in]
                n215 = call "LogEngine.LogFile.Convert.vi"("error in (no error)"=w582, "path"=w583) -> ("error out"=w586:errorcluster, "Status"=w589:string)  [unwired: 8 in]
                n216 = property class="Str"(reference=w585, "Value"=w589) -> (error out=w587:errorcluster)  [unwired: 1 in, 1 out]
                n217 = Merge Errors(w587, w586) -> (w584:errorcluster)
              }
            }
          }
          frame True {
            # "No open log file. Do nothing."
          }
        }
        n218 = Equal?(x=SubProcessEngine.State."Exit", y=w567) -> (x = y?=w571:bool)
        n219 = Select(t=w567, s=w571, f=SubProcessEngine.State."Idle" ("x")) -> (s? t:f=w568:T7)
      }
    }
  }
  n220 = while {
    tunnel: w18 -> [w613]
    tunnel: w17 -> [w615]
    tunnel: [w614] -> w9
    shift-right: [w612] -> _
    shift-left: SubProcessEngine.State."Idle" ("State") -> [w607]
    tunnel: w10 -> [w611]
    shift-right: [w609] -> _
    shift-left: _ -> [w595]
    stop <- w608 stop-if-true
    # "Process Results Loop - Process the Bus Data/Status from the gRPC Stream loop based on User parameters and display results."
    n221 = call "SubProcessEngine.GetNextState.vi"("error in (no error)"=w611, "State"=w607, "timeout in ms (5)"=250, "Q"=w613) -> ("error out"=w597:errorcluster, "State"=w593:T7, "timed out?"=w606:bool, "Data"=w610:T34)  [unwired: 4 in]
    n222 = flat-sequence {
      tunnel: ["Pause"] -> w604
      tunnel: ["Type Filter"] -> w603
      tunnel: ["Direction Filter"] -> w602
      tunnel: ["Host Filter"] -> w601
      tunnel: ["Filter IDs"] -> w600
      tunnel: ["Clear History"] -> w599
      tunnel: ["Sort By ID"] -> w598
      tunnel: w597 -> [w619]
      tunnel: [w619] -> w596
      tunnel: w595 -> [w618]
      tunnel: [w618] -> w594
      tunnel: w593 -> [w617]
      tunnel: [w617] -> w592
      frame #0 {
      }
    }
    n223 = case shown="\"Process\"" w592 {
      selector: w592 -> [w633 _ _ _ w689]
      tunnel: w615 -> [w629 _ w664 w680 w684]
      tunnel: [w627 w634 w646 w675 w682] -> w614
      tunnel: [w633 SubProcessEngine.State."Process" ("State") SubProcessEngine.State."Process" ("State") SubProcessEngine.State."Idle" ("State") w689] -> w612
      tunnel: w596 -> [w628 w634 w660 w677 w683]
      tunnel: w610 -> [_ _ w662 _ _]
      tunnel: [_ TRUE _ _ _] -> w609
      tunnel: w594 -> [_ _ w650 _ _]
      tunnel: [_ _ _ _ TRUE] -> w608
      tunnel: w606 -> [_ _ w656 _ _]
      tunnel: w604 -> [_ _ w645 _ _]
      tunnel: w603 -> [_ _ w644 _ _]
      tunnel: w602 -> [_ _ w643 _ _]
      tunnel: w601 -> [_ _ w642 _ _]
      tunnel: w600 -> [_ _ w641 _ _]
      tunnel: w599 -> [_ _ w640 _ _]
      tunnel: w598 -> [_ _ w639 _ _]
      tunnel: [_ _ w638 _ _] -> w591
      tunnel: [_ _ w637 _ _] -> w590
      frame "Idle" {
        # "Do Nothing."
        n224 = property class="Str"(reference=w629, "Value"="Bus: Idle..", "Blinking"=FALSE) -> (error out=w630:errorcluster)  [unwired: 1 in, 1 out]
        n225 = Merge Errors(w630, w628) -> (w627:errorcluster)
      }
      frame "Arm" {
        # "Set the re-init flag and go to the next state."
      }
      frame "Process" {
        # "Handle bus data. Allowing timeouts is required so user parameters are applied, even if new data is not available."
        n226 = Unbundle By Name(w662) -> ("Parameters"=w661:variant)
        n227 = call "Convert.StringToArray.vi"("Filter IDs"=w641) -> ("Filter IDs"=w654:u32[])  [unwired: 10 in]
        n228 = Variant To Data(error in=w660, type=T29 {"Response Data"={"can_comm_state"={"fault_code"=0, "fault"=FALSE, "comm_state"=enum."Error_Active", "last_comm_error"=enum."None", "receive_error_counter"=0, "transmit_error_counter"=0, "transceiver_error"=FALSE, "sleep"=FALSE}, "frame"=[], "error"={"status"=FALSE, "code"=0, "source"=""}}, "Success"=FALSE} ("cluster"), Variant=w661) -> (data=w659:T29, error out=w649:errorcluster)
        n229 = Bundle By Name(cluster=T36 {"Host Filter"=FALSE, "Filter Parameters"={"filter_ids"=[], "direction_filter"=enum."TX_RX", "frame_filter"=enum."CAN_Data"}, "Sort By ID"=FALSE, "Pause"=FALSE, "Clear History"=FALSE} ("Host Parameters"), "Clear History"=w640, "Pause"=w645, "Sort By ID"=w639, "Filter Parameters.direction_filter"=w643, "Filter Parameters.frame_filter"=w644, "Host Filter"=w642, "Filter Parameters.filter_ids"=w654) -> (w651:T36)
        n230 = Unbundle By Name(w659) -> ("Response Data.can_comm_state"=w657:T31, "Success"=w652:bool, "Response Data.frame"=w658:T16[])
        n231 = case shown="False" w656 {
          tunnel: w664 -> [w673 _]
          tunnel: [w669 w674] -> w648
          tunnel: w657 -> [w668 _]
          tunnel: w652 -> [w666 _]
          tunnel: w649 -> [w665 w674]
          frame False {
            # "Process Comm State"
            n232 = call "StreamEngine.Main.Stream.BusStatus.Process.vi"("error in (no error)"=w665, "Stream Connection"=w666, "State"=w668) -> ("error out"=w670:errorcluster, "Warning"=w672:bool, "State"=w667:string)  [unwired: 6 in]
            n233 = property class="Str"(reference=w673, "Value"=w667, "Blinking"=w672) -> (error out=w671:errorcluster)  [unwired: 1 in, 1 out]
            n234 = Merge Errors(w671, w670) -> (w669:errorcluster)
          }
          frame True {
            # "Timeout. Do nothing."
          }
        }
        n235 = call "StreamEngine.Main.Stream.BusData.Process.vi"("error in (no error)"=w649, "Host Parameters"=w651, "Init?"=w650, "frame"=w658) -> ("error out"=w647:errorcluster, "Table Update"=w638:bool, "Table"=w637:string[][])  [unwired: 5 in]
        n236 = Merge Errors(w648, w647) -> (w646:errorcluster)
      }
      frame "Stop" {
        # "Stop the data processing loop."
        n237 = property class="Str"(reference=w680, "Value"="Bus: Stopping..", "Blinking"=FALSE) -> (error out=w676:errorcluster)  [unwired: 1 in, 1 out]
        n238 = Merge Errors(w676, w677) -> (w675:errorcluster)
      }
      frame "Exit" {
        # "Exit the data processing loop."
        n239 = property class="Str"(reference=w684, "Value"="Bus: Exiting..", "Blinking"=FALSE) -> (error out=w685:errorcluster)  [unwired: 1 in, 1 out]
        n240 = Merge Errors(w685, w683) -> (w682:errorcluster)
      }
    }
    n241 = case shown="True" w591 {
      tunnel: w590 -> [_ w616]
      frame False {
      }
      frame True {
        "Table Control" <- w616
      }
    }
  }
  n242 = while {
    shift-right: [w699] -> _
    shift-left: StreamEngine.State."Wait" -> [w691]
    tunnel: w10 -> [w700]
    shift-right: [w698] -> _
    shift-left: T5 0 ("Call ID") -> [w697]
    tunnel: w20 -> [w695]
    tunnel: [w694] -> w19
    tunnel: w15 -> [w692]
    stop <- w696 stop-if-true
    # "gRPC Stream Loop - Begin, Read, and End the gRPC Stream for Bus Data/Status"
    n243 = call "StreamEngine.GetNextStreamState.vi"("error in (no error)"=w700, "Bus State"=w691, "Cmd Q"=w695) -> ("error out"=w701:errorcluster, "Bus State"=w690:T8, "Command Cluster"=w702:T37)  [unwired: 5 in, 1 out]
    n244 = case shown="\"Start Stream\"" w690 {
      selector: w690 -> [w703 _ w721 _ w732]
      tunnel: w701 -> [w704 w707 w718 w727 w734]
      tunnel: w702 -> [_ w710 _ _ _]
      tunnel: [w704 w708 w716 w725 w731] -> w694
      tunnel: [_ w709 w717 _ _] -> w698
      tunnel: w697 -> [_ _ w719 w726 w733]
      tunnel: [w703 w711 w720 StreamEngine.State."Wait" w732] -> w699
      tunnel: [_ _ _ w724 w730] -> w696
      tunnel: [_ _ w715 _ _] -> w693
      tunnel: w692 -> [_ w706 w714 w723 w729]
      frame "Wait", Default {
        # "Do Nothing"
      }
      frame "Start Stream" {
        # "Begin gRPC Stream"
        n245 = Unbundle By Name(w710) -> ("Parameters"=w705:variant)
        n246 = call "StreamEngine.Main.Stream.Start.vi"("Stream.Qs.SubProcesses"=w706, "error in (no error)"=w707, "Parameters"=w705) -> ("error out"=w708:errorcluster, "Stream Ref"=w709:T5)  [unwired: 6 in, 1 out]
        n247 = Select(t=StreamEngine.State."Stop Stream", s=w708, f=StreamEngine.State."Read Stream") -> (s? t:f=w711:T8)
      }
      frame "Read Stream" {
        # "Read Data from gRPC Stream"
        n248 = call "StreamEngine.Main.Stream.Read.vi"("error in (no error)"=w718, "SubProcesses"=w714, "gRPC ID"=w719) -> ("error out"=w716:errorcluster, "Success"=w715:bool, "gRPC ID out"=w717:T5)  [unwired: 6 in]
        n249 = Select(t=StreamEngine.State."Stop Stream", s=w716, f=w721) -> (s? t:f=w720:T8)
      }
      frame "Stop Stream" {
        w724 = FALSE ("Exit?")
        # "Close gRPC Stream"
        n250 = call "StreamEngine.Main.Stream.Stop.vi"("error in (no error)"=w727, "Exit?"=w724, "Stream.Qs.SubProcesses"=w723, "Stream Ref"=w726) -> ("error out"=w725:errorcluster)  [unwired: 7 in]
      }
      frame "Exit" {
        w730 = TRUE
        # "Exit Loop"
        n251 = call "StreamEngine.Main.Stream.Stop.vi"("error in (no error)"=w734, "Exit?"=w730, "Stream.Qs.SubProcesses"=w729, "Stream Ref"=w733) -> ("error out"=w731:errorcluster)  [unwired: 7 in]
      }
    }
    "Stream Connected" <- w693
  }
  n252 = flat-sequence {
    tunnel: w43 -> [w740]
    tunnel: w19 -> [w738]
    tunnel: w9 -> [w737]
    tunnel: w8 -> [w739]
    tunnel: w7 -> [w736]
    tunnel: [w735] -> w1
    tunnel: [w741] -> w2
    tunnel: w1 -> [w741]
    frame #0 {
      n253 = call "GUI.Close.vi"("State Variables in"=w740) -> ()  [unwired: 11 in]
      n254 = Merge Errors(w739, w738, w737, w736) -> (w735:errorcluster)
    }
    frame #1 {
      n255 = invoke class="VI" method="FP.Close"() -> ()  [unwired: 3 in, 3 out]
    }
  }
  "error out" <- w2
